vi "set_bias_0.vi"() -> ()   [LabVIEW 2014]
uses:
  <userlib>/Nanonis Prog Interface V5/Nanonis Prog Interface.lvlib
panel:
  in  "milliseconds to wait":u32=800
  out "Status":string
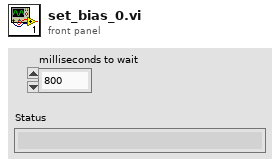
[diagram p1: front panel]
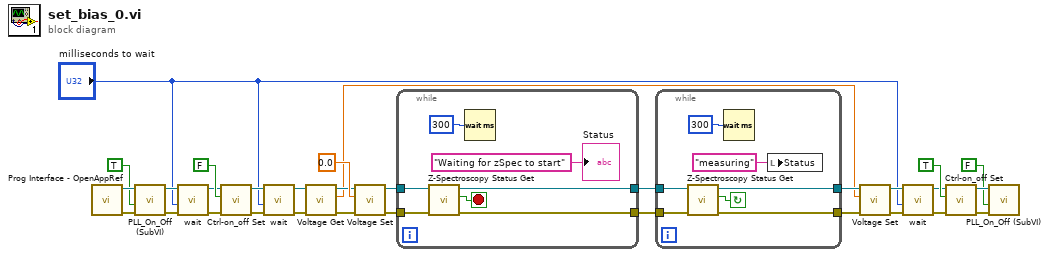
[diagram p0: block diagram]
diagram:
  n1 = call <userlib>:"Prog Interface - OpenAppRef.vi"() -> ("Error out"=w31:errorcluster, "Application reference"=w30:refnum<vi>)  [unwired: 6 in]
  n2 = call "PLL_On_Off (SubVI).vi"("error in (no error)"=w31, "Output ON/OFF (F=OFF)"=TRUE, "Application in"=w30) -> ("error out"=w13:errorcluster, "Application out"=w7:refnum<vi>)  [unwired: 7 in]
  n3 = call "wait.vi"("error in"=w13, "milliseconds to wait"="milliseconds to wait", "application reference in"=w7) -> ("error out"=w12:errorcluster, "application reference out"=w6:refnum<vi>)  [unwired: 7 in]
  n4 = call <userlib>:"Ctrl-on_off Set.vi"("error in (no error)"=w12, "Z Controller ON/OFF"=FALSE, "Application ref in"=w6) -> ("error out"=w11:errorcluster, "Application ref out"=w8:refnum<vi>)  [unwired: 7 in]
  n5 = call "wait.vi"("error in"=w11, "milliseconds to wait"="milliseconds to wait", "application reference in"=w8) -> ("error out"=w10:errorcluster, "application reference out"=w9:refnum<vi>)  [unwired: 7 in]
  n6 = call <userlib>:"Voltage Get.vi"("error in (no error)"=w10, "Application ref in"=w9) -> ("error out"=w19:errorcluster, "Bias (V)"=w18:sgl, "Application ref out"=w20:refnum<vi>)  [unwired: 7 in]
  n7 = call <userlib>:"Voltage Set.vi"("Error in (no error)"=w19, "Bias (V)"=sgl 0.0, "Application ref in"=w20) -> ("Error out"=w26:errorcluster, "Application ref out"=w25:refnum<vi>)  [unwired: 7 in]
  n8 = while {
    tunnel: w26 -> [w38]
    tunnel: w25 -> [w37]
    tunnel: [w34] -> w24
    tunnel: [w33] -> w23
    stop <- w36 stop-if-true
    n9 = call <userlib>:"Z-Spectroscopy Status Get.vi"("Error in (no error)"=w38, "Application ref in"=w37) -> ("Error out"=w33:errorcluster, "Running?"=w36:bool, "Application ref out"=w34:refnum<vi>)  [unwired: 5 in]
    n10 = Wait (ms)(milliseconds to wait=u32 300) -> ()  [unwired: 1 out]
    "Status" <- "Waiting for zSpec to start" ("Status")
  }
  n11 = while {
    tunnel: w24 -> [w43]
    tunnel: w23 -> [w42]
    tunnel: [w41] -> w22
    tunnel: [w40] -> w21
    stop <- w45 continue-if-true
    n12 = call <userlib>:"Z-Spectroscopy Status Get.vi"("Error in (no error)"=w42, "Application ref in"=w43) -> ("Error out"=w40:errorcluster, "Running?"=w45:bool, "Application ref out"=w41:refnum<vi>)  [unwired: 5 in]
    n13 = Wait (ms)(milliseconds to wait=u32 300) -> ()  [unwired: 1 out]
    n14 = local write "Status"("measuring" ("Status")) -> ()
  }
  n15 = call <userlib>:"Voltage Set.vi"("Error in (no error)"=w21, "Bias (V)"=w18, "Application ref in"=w22) -> ("Error out"=w4:errorcluster, "Application ref out"=w5:refnum<vi>)  [unwired: 7 in]
  n16 = call "wait.vi"("error in"=w4, "milliseconds to wait"="milliseconds to wait", "application reference in"=w5) -> ("error out"=w3:errorcluster, "application reference out"=w2:refnum<vi>)  [unwired: 7 in]
  n17 = call <userlib>:"Ctrl-on_off Set.vi"("error in (no error)"=w3, "Z Controller ON/OFF"=TRUE, "Application ref in"=w2) -> ("error out"=w15:errorcluster, "Application ref out"=w16:refnum<vi>)  [unwired: 7 in]
  n18 = call "PLL_On_Off (SubVI).vi"("error in (no error)"=w15, "Output ON/OFF (F=OFF)"=FALSE, "Application in"=w16) -> ()  [unwired: 7 in, 2 out]
